vi "Start Main.vi"(6 "시트잠금?":refnum<vi>, 8 "에러 입력(에러 없음)":errorcluster, 9 "교정절차 목록 MC List":refnum<vi>, 10 "교정환경":refnum<vi>, 11 "교정정보":refnum<vi>) -> (0 "에러 출력":errorcluster, 3 "큐 출력":refnum<queue>, 4 "출력 클러스터":T1={"경로"=path "", "Version"="", "상태"=enum."Maximized", "기준기정렬"=0, "창높이"=0, "창넓이"=0}, 5 "이벤트 등록 참조 번호 출력":refnum<event-registration>, 7 "사용자 이벤트 - 정지":refnum<user-event>)   [LabVIEW 2020]
uses:
  Controls/Message Cluster.ctl
  Controls/Clst_Atm Info Main.ctl
  Controls/Clst_Cal Info Main.ctl
  Controls/Clst_Cal Info Global.ctl
  Controls/Cmd_Read Query.ctl
  Variables/Global_Cal Info.vi
  Public/Polymorph/ini Ctrl_1D Str.vi
  <vilib>/addons/database/NI_Database_API.lvlib
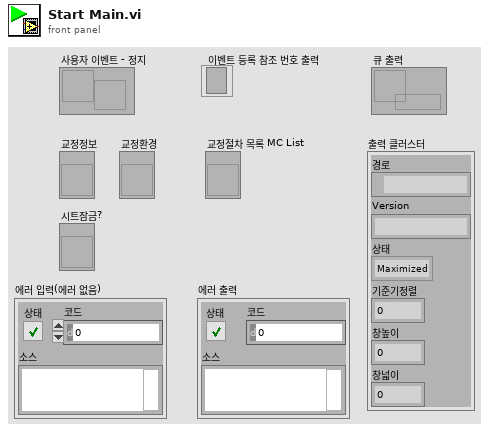
[diagram p1: front panel]
types:
  T1 = cluster{"경로":path, "Version":string, "상태":enum32{"Invalid", "Standard", "Closed", "Hidden", "Minimized", "Maximized"}, "기준기정렬":u16, "창높이":u32, "창넓이":u32}
  T2 = typedef "Cmd_Read Query.ctl" = enum16{"교정자 이름 얻기", "인증교정자 얻기", "기술책임자 얻기", "기책부책 얻기", "등록번호 얻기", "등록정보 얻기", "업체정보 얻기", "교정일자(CAMAS) 얻기", "교정일자(CALSTD) 얻기", "교정환경 얻기", "교정절차서 목록 얻기", "교정절차서명 얻기", "교정절차 목록얻기", "교정절차 얻기", "PROC 교정절차 얻기", "PROC SPEC 얻기", "교정절차(Func별) 얻기", "교정절차(Func_ext별) 얻기", "기관코드 얻기", "교정기능(세부분류) 얻기", "교정기능(모델) 얻기", "교정기능 목록 얻기", "교정기능 명칭 얻기", "교정기능 항목명칭 얻기", "DB (사용기준기) 얻기", "DB (기준기이름) 얻기", "DB (기준기이름목록) 얻기", "DB (기준기목록) 얻기", "DB (기준기값) 얻기", "DB (CMC) 얻기", "DB (FUNC) 얻기", "DB (CALNAME) 얻기", "DB (STDNAME) 얻기", "DB (SPEC) 얻기", "모델(항목전체) 얻기", "모델(최대범위) 얻기", "모델(최소범위) 얻기", "모델(최대최소) 얻기", "모델(범위조건) 얻기", "모델(등록요청) 얻기", "모델(형식별) 얻기", "모델(조건별) 얻기", "모델(모델검색) 얻기", "세부분류 목록 얻기", "기준기등록리스트 얻기", "STD Cal Date Check", "DB등록일자 얻기", "적용항목 얻기", "기타정보 얻기", "기준기요청 얻기", "서버버전 얻기"}
  T3 = cluster{"세부분류코드":string, "형식":string, "옵션":string, "측정기명":string, "측정기명 2":string, "세부분류코드 2":string}
  T4 = typedef "Clst_Atm Info Main.ctl" = cluster{"교정장소":enum16{"0 : 고정표준실", "1 : 현장교정"}, "최저온도(℃)":string, "최고온도(℃)":string, "최저습도(％ R.H.)":string, "최고습도(％ R.H.)":string, "최저기압(hPa)":string, "최고기압(hPa)":string, "교정실명":string}
  T5 = typedef "Clst_Cal Info Global.ctl" = cluster{"등록번호":string, "의뢰기관":string, "기기명":string, "제작회사":string, "형식":string, "기기번호":string, "소분류코드":string, "세부분류코드":string, "교정주기":string, "접수번호":string, "교정일자":string, "교정절차서 1":string, "교정절차서 2":string, "교정절차서 3":string, "접수확인자":string, "인증교정자":string, "기술책임자":string, "KOLAS 유무":string, "진행상태":string, "의뢰기관코드":string, "입고형태":string, "영문성적서?":bool, "합불판정?":bool, "부록?":bool, "절차서번호 1":string, "절차서번호 2":string, "절차서번호 3":string, "교정방식":string, "부서명":string}
  T6 = enum32{"invalid app kind", "Development System", "Run Time System", "Student Edition", "Embedded LabVIEW", "Evaluation", "Custom"}
  T7 = typedef "NI_Database_API.lvlib/Conn ObjectReference.ctl" = refnum<k1>
  T8 = enum32{"Invalid", "Standard", "Closed", "Hidden", "Minimized", "Maximized"}
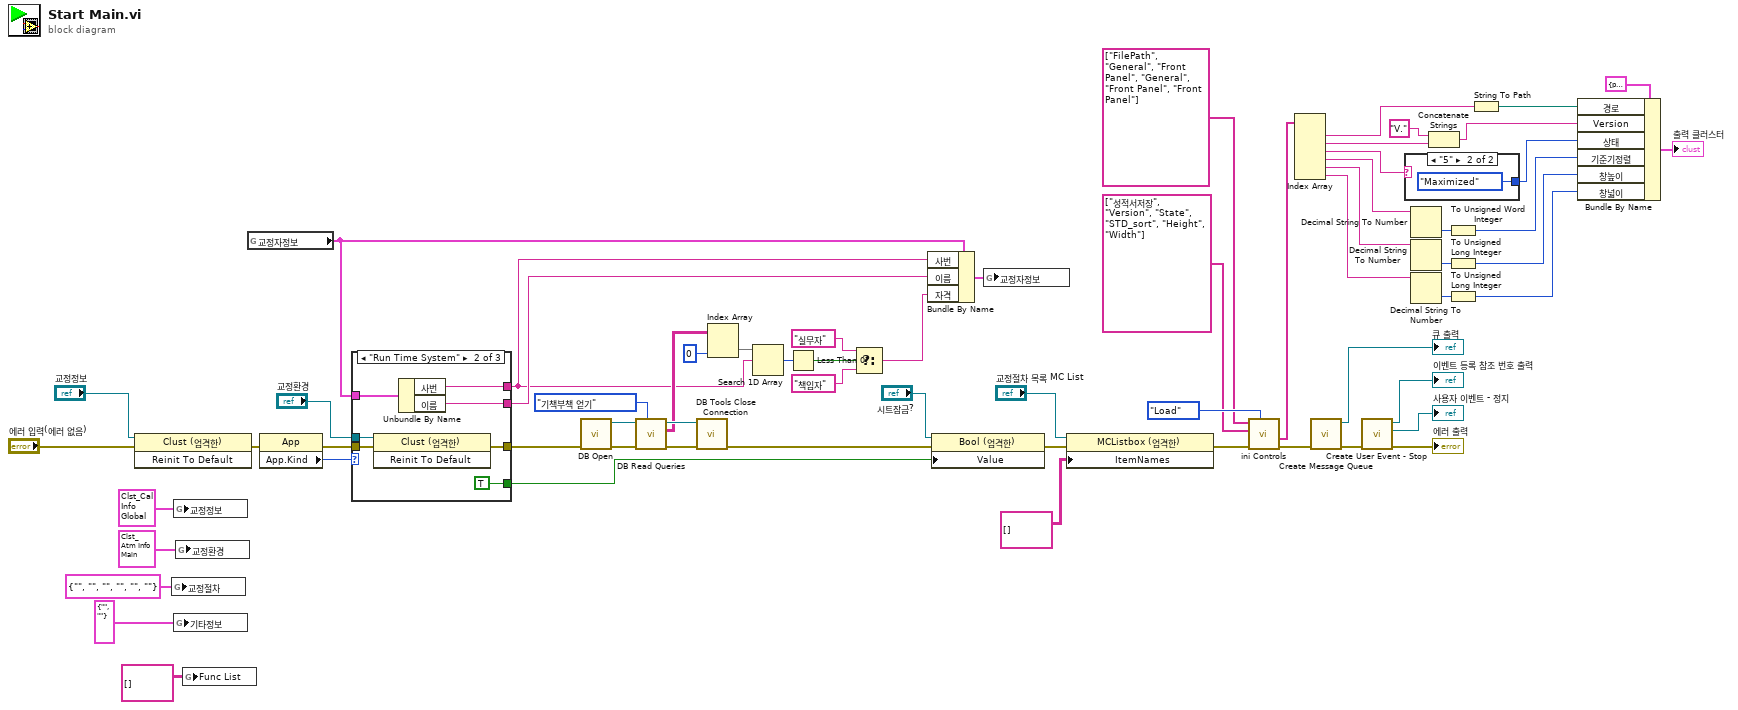
[diagram p0: block diagram]
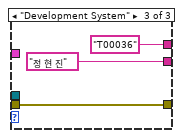
[diagram p3: hidden frame]
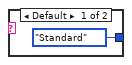
[diagram p4: hidden frame]
diagram:
  n1 = invoke class="Clust (엄격한)" method="Reinit To Default"(reference="교정정보", error in="에러 입력(에러 없음)") -> (error out=w44:errorcluster)  [unwired: 1 in, 2 out]
  n2 = global write "Global_Cal Info.vi" "교정절차"(T3 {"세부분류코드"="", "형식"="", "옵션"="", "측정기명"="", "측정기명 2"="", "세부분류코드 2"=""} ("교정절차")) -> ()
  n3 = global write "Global_Cal Info.vi" "교정정보"(T5 {"등록번호"="", "의뢰기관"="", "기기명"="", "제작회사"="", "형식"="", "기기번호"="", "소분류코드"="", "세부분류코드"="", "교정주기"="", "접수번호"="", "교정일자"="", "교정절차서 1"="", "교정절차서 2"="", "교정절차서 3"="", "접수확인자"="", "인증교정자"="", "기술책임자"="", "KOLAS 유무"="", "진행상태"="", "의뢰기관코드"="", "입고형태"="", "영문성적서?"=FALSE, "합불판정?"=FALSE, "부록?"=FALSE, "절차서번호 1"="", "절차서번호 2"="", "절차서번호 3"="", "교정방식"="", "부서명"=""} ("교정정보")) -> ()
  n4 = global write "Global_Cal Info.vi" "기타정보"(cluster{"부서코드":string, "제조사코드":string} {"부서코드"="", "제조사코드"=""} ("기타정보")) -> ()
  n5 = global write "Global_Cal Info.vi" "교정환경"(T4 {"교정장소"=enum."0 : 고정표준실", "최저온도(℃)"="", "최고온도(℃)"="", "최저습도(％ R.H.)"="", "최고습도(％ R.H.)"="", "최저기압(hPa)"="", "최고기압(hPa)"="", "교정실명"=""} ("교정환경")) -> ()
  n6 = global write "Global_Cal Info.vi" "Func List"(string[][] [] ("Func List")) -> ()
  n7 = global read "Global_Cal Info.vi" "교정자정보"() -> (w10:cluster{"사번":string, "이름":string, "자격":string})
  n8 = property class="App"(error in=w44) -> (error out=w43:errorcluster, "App.Kind"=w45:T6)  [unwired: 1 in, 1 out]
  n9 = case shown="\"Run Time System\"" w45 {
    tunnel: w43 -> [w65 w72 w75]
    tunnel: [w65 w69 w75] -> w13
    tunnel: "교정환경" -> [_ w71 _]
    tunnel: [_ TRUE _] -> w23
    tunnel: w10 -> [_ w68 _]
    tunnel: [_ w67 "T00036" ("사번")] -> w3
    tunnel: [_ w66 "정 현 진" ("이름")] -> w9
    frame Default {
    }
    frame "Run Time System" {
      n10 = invoke class="Clust (엄격한)" method="Reinit To Default"(reference=w71, error in=w72) -> (error out=w69:errorcluster)  [unwired: 1 in, 2 out]
      n11 = Unbundle By Name(w68) -> ("사번"=w67:string, "이름"=w66:string)
    }
    frame "Development System" {
    }
  }
  n12 = call "DB Open.vi"("에러 입력"=w13) -> ("에러 출력"=w18:errorcluster, "참조 번호 출력"=w17:T7)  [unwired: 9 in]
  n13 = call "DB Read Queries.vi"("Query Command"=Cmd_Read_Query."기책부책 얻기", "에러 입력(에러 없음)"=w18, "참조 번호 입력"=w17) -> ("에러 출력"=w19:errorcluster, "Data"=w5:string[][], "참조 번호 출력"=w16:T7)  [unwired: 4 in, 2 out]
  n14 = call <vilib>:"DB Tools Close Connection.vi"("error in (no error)"=w19, "connection reference"=w16) -> ("error out"=w12:errorcluster)  [unwired: 5 in]
  n15 = Index Array(array=w5, index (col)=0 ("비활성화된 인덱스 (열)")) -> (element=w2:string[])  [unwired: 1 in]
  n16 = Search 1D Array(1D array=w2, element=w3) -> (index of element=w1:i32)  [unwired: 1 in]
  n17 = Less Than 0?(x=w1) -> (x < 0?=w8:bool)
  n18 = Select(t="실무자", s=w8, f="책임자") -> (s? t:f=w4:string)
  n19 = Bundle By Name(cluster=w10, "사번"=w3, "이름"=w9, "자격"=w4) -> (w20:cluster{"사번":string, "이름":string, "자격":string})
  n20 = property class="Bool (엄격한)"(reference="시트잠금?", error in=w12, "Value"=w23) -> (error out=w11:errorcluster)  [unwired: 1 out]
  n21 = global write "Global_Cal Info.vi" "교정자정보"(w20) -> ()
  n22 = property class="MCListbox (엄격한)"(reference="교정절차 목록 MC List", error in=w11, "ItemNames"=string[][] [] ("아이템 이름")) -> (error out=w54:errorcluster)  [unwired: 1 out]
  n23 = call-poly "ini Controls.vi"("Select"=enum16{"Save", "Load"}."Load", "에러 입력"=w54, "키"=string[] ["성적서저장", "Version", "State", "STD_sort", "Height", "Width"], "섹션"=string[] ["FilePath", "General", "Front Panel", "General", "Front Panel", "Front Panel"]) -> ("에러 출력"=w29:errorcluster, "값"=w47:string[])  [unwired: 5 in, 1 out]
  n24 = Index Array(array=w47) -> (element #1=w49:string, element #2=w48:string, element #3=w46:string, element #4=w42:string, element #5=w34:string, element #6=w33:string)  [unwired: 6 in]
  n25 = call "Create Message Queue.vi"("에러 입력(에러 없음)"=w29) -> ("에러 출력"=w62:errorcluster, "큐 출력"=→"큐 출력":refnum<queue>)  [unwired: 9 in]
  n26 = call "Create User Event - Stop.vi"("에러 입력(에러 없음)"=w62) -> ("에러 출력"=→"에러 출력":errorcluster, "사용자 이벤트 - 정지"=→"사용자 이벤트 - 정지":refnum<user-event>, "이벤트 등록 참조 번호 출력"=→"이벤트 등록 참조 번호 출력":refnum<event-registration>)  [unwired: 8 in]
  n27 = case shown="\"5\"" w46 {
    tunnel: [T8."Standard" ("프런트패널 윈도우:상태") T8."Maximized" ("프런트패널 윈도우:상태")] -> w27
    frame Default {
    }
    frame "5" {
    }
  }
  n28 = Decimal String To Number(string=w42) -> (number=w41:i32)  [unwired: 2 in, 1 out]
  n29 = Decimal String To Number(string=w34) -> (number=w36:i32)  [unwired: 2 in, 1 out]
  n30 = Decimal String To Number(string=w33) -> (number=w35:i32)  [unwired: 2 in, 1 out]
  n31 = Concatenate Strings("V." ("문자열"), w48) -> (w39:string)
  n32 = To Unsigned Word Integer(number=w41) -> (unsigned 16bit integer=w38:u16)
  n33 = To Unsigned Long Integer(number=w36) -> (unsigned 32bit integer=w32:u32)
  n34 = To Unsigned Long Integer(number=w35) -> (unsigned 32bit integer=w31:u32)
  n35 = String To Path(string=w49) -> (path=w40:path)
  n36 = Bundle By Name(cluster=T1 {"경로"=path "", "Version"="", "상태"=enum."Invalid", "기준기정렬"=0, "창높이"=0, "창넓이"=0}, "경로"=w40, "Version"=w39, "상태"=w27, "기준기정렬"=w38, "창높이"=w32, "창넓이"=w31) -> (→"출력 클러스터":T1)
